vi "array -- bilinear regression 3D -- V3.vi"(7 "action":T3, 9 "fit map IN":map{T2, dbl}(c390), 11 "xyzw IN":T1={"x"=[-2.0, -1.0, 0.0, 1.0, 2.0], "y"=[-2.0, -1.0, 0.0, 1.0, 2.0], "w"=[-2.0, -1.0, 0.0, 1.0, 2.0], "z"=[12.0, 3.0, 0.0, 3.0, 12.0]}) -> (1 "fit map out":map{T2, dbl}(c390), 3 "xyzw OUT":T1={"x"=[-2.0, -1.0, 0.0, 1.0, 2.0], "y"=[-2.0, -1.0, 0.0, 1.0, 2.0], "w"=[-2.0, -1.0, 0.0, 1.0, 2.0], "z"=[12.0, 3.0, 0.0, 3.0, 12.0]})   [LabVIEW 2021]
uses:
  array -- fit control .ctl
  array -- bilinear regression 2D.ctl
  4-vec-array.ctl
  <vilib>/Analysis/baseanly.llb/Matrix Type of Inverse Matrix.ctl
  <vilib>/Analysis/7linalg.llb/Solve Linear Equations (single right hand).vi
  <vilib>/Analysis/baseanly.llb/Real A x B.vi
  <vilib>/Analysis/baseanly.llb/Solve Linear Equations By Cholesky.vi
  <vilib>/Analysis/baseanly.llb/Real Matrix to Compact Array.vi
  <vilib>/Analysis/baseanly.llb/Real Compact Tri-Matrix Linear Eqs.vi
  <vilib>/Analysis/Matrix/Numeric/Conversions/Array To Matrix - RA2.vi
  <vilib>/Analysis/7linalg.llb/Solve Linear Eqs (General).vi
  <vilib>/Analysis/7linalg.llb/Solve Linear Eqs (Gen, single right hand).vi
  <vilib>/Analysis/Matrix/Numeric/Conversions/Matrix To Array - RM.vi
  <vilib>/Analysis/NI_AALBase.lvlib
  <vilib>/Analysis/Matrix/NI_Matrix.lvlib
  <vilib>/Analysis/NI_AALPro.lvlib
panel:
  out "fit  IN":dbl[](array[numeric])=[1.9, 2.6, 3.3, 1.0, 2.7, 3.9]
  out "fit OUT":dbl[](array[numeric])=[1.0, 1.0, 1.0, 0.0, 0.0, 0.0]
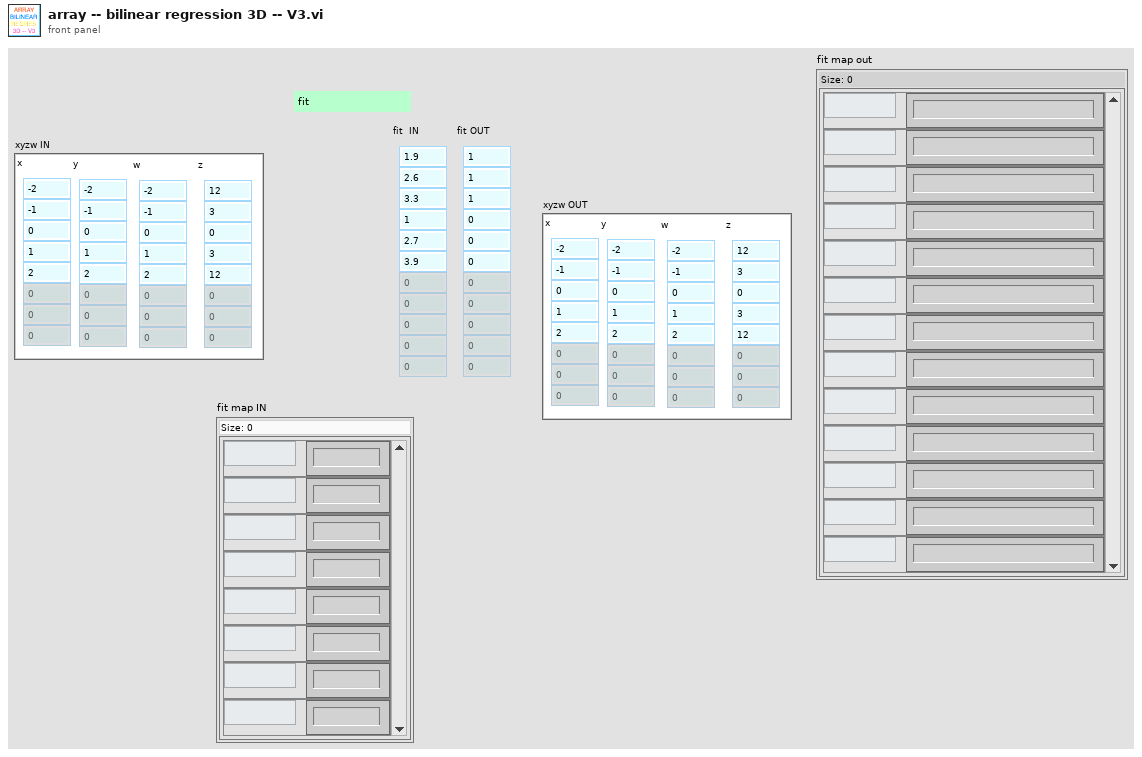
[diagram p1: front panel]
types:
  T1 = typedef "4-vec-array.ctl" = cluster{"x":dbl[], "y":dbl[], "w":dbl[], "z":dbl[]}
  T2 = typedef "array -- bilinear regression 2D.ctl" = enum16{"1", "x", "y", "xx", "xy", "yy", "xxy", "xyy", "yyy", "xxx", "xxyy", "xyyy", "xxxy", "yyyy", "xxxx", "xxz", "xyz", "yyz", "xz", "yz", "z", "wwz", "ywz", "xwz", "xxxw", "xxyw", "xyyw", "yyyw", "xxww", "xyww", "yyww", "xwww", "ywww", "wwww", "ww", "xw", "yw", "w", "wz", "xxw", "yyw", "xyw", "xww", "yww", "www"}
  T3 = typedef "array -- fit control .ctl" = enum16{"fit", "calc", "check", "init"}
  T4 = typedef "NI_AALBase.lvlib/Matrix Type of Inverse Matrix.ctl" = enum32{"General", "Positive Definite", "Lower Triangular", "Upper Triangular"}
  T5 = typedef "NI_Matrix.lvlib/RealMatrix.ctl" = dbl[][]
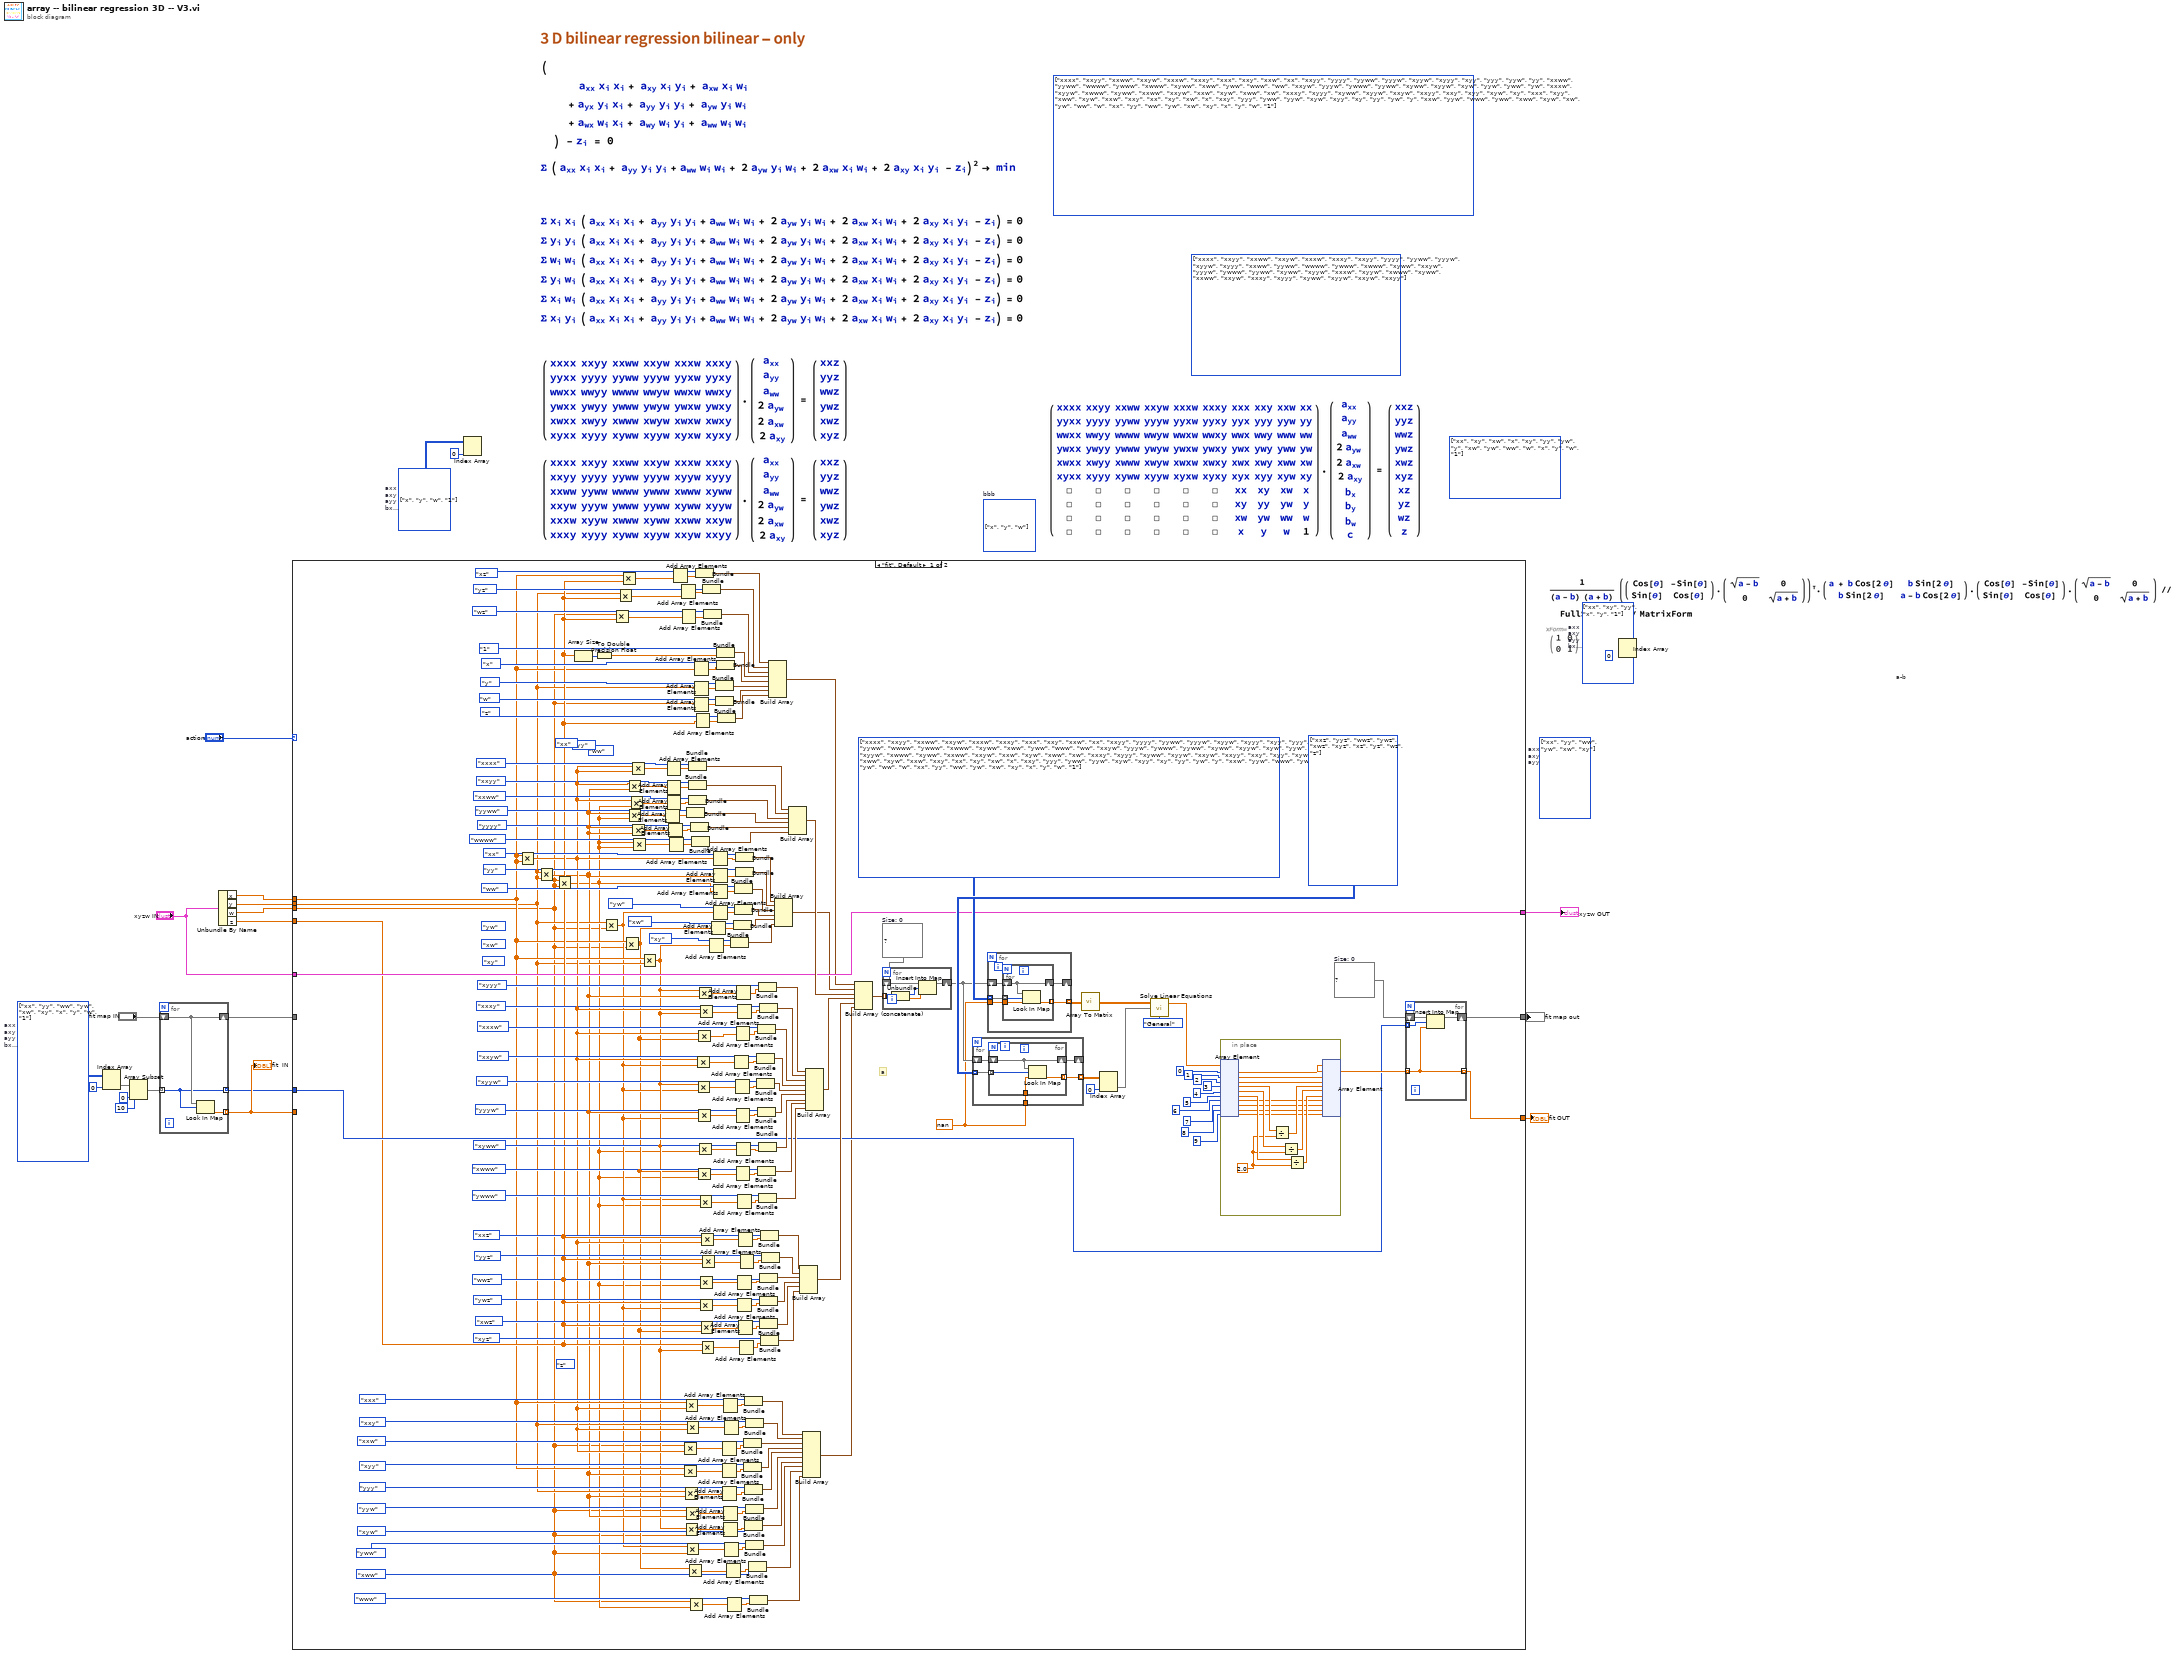
[diagram p0: block diagram]
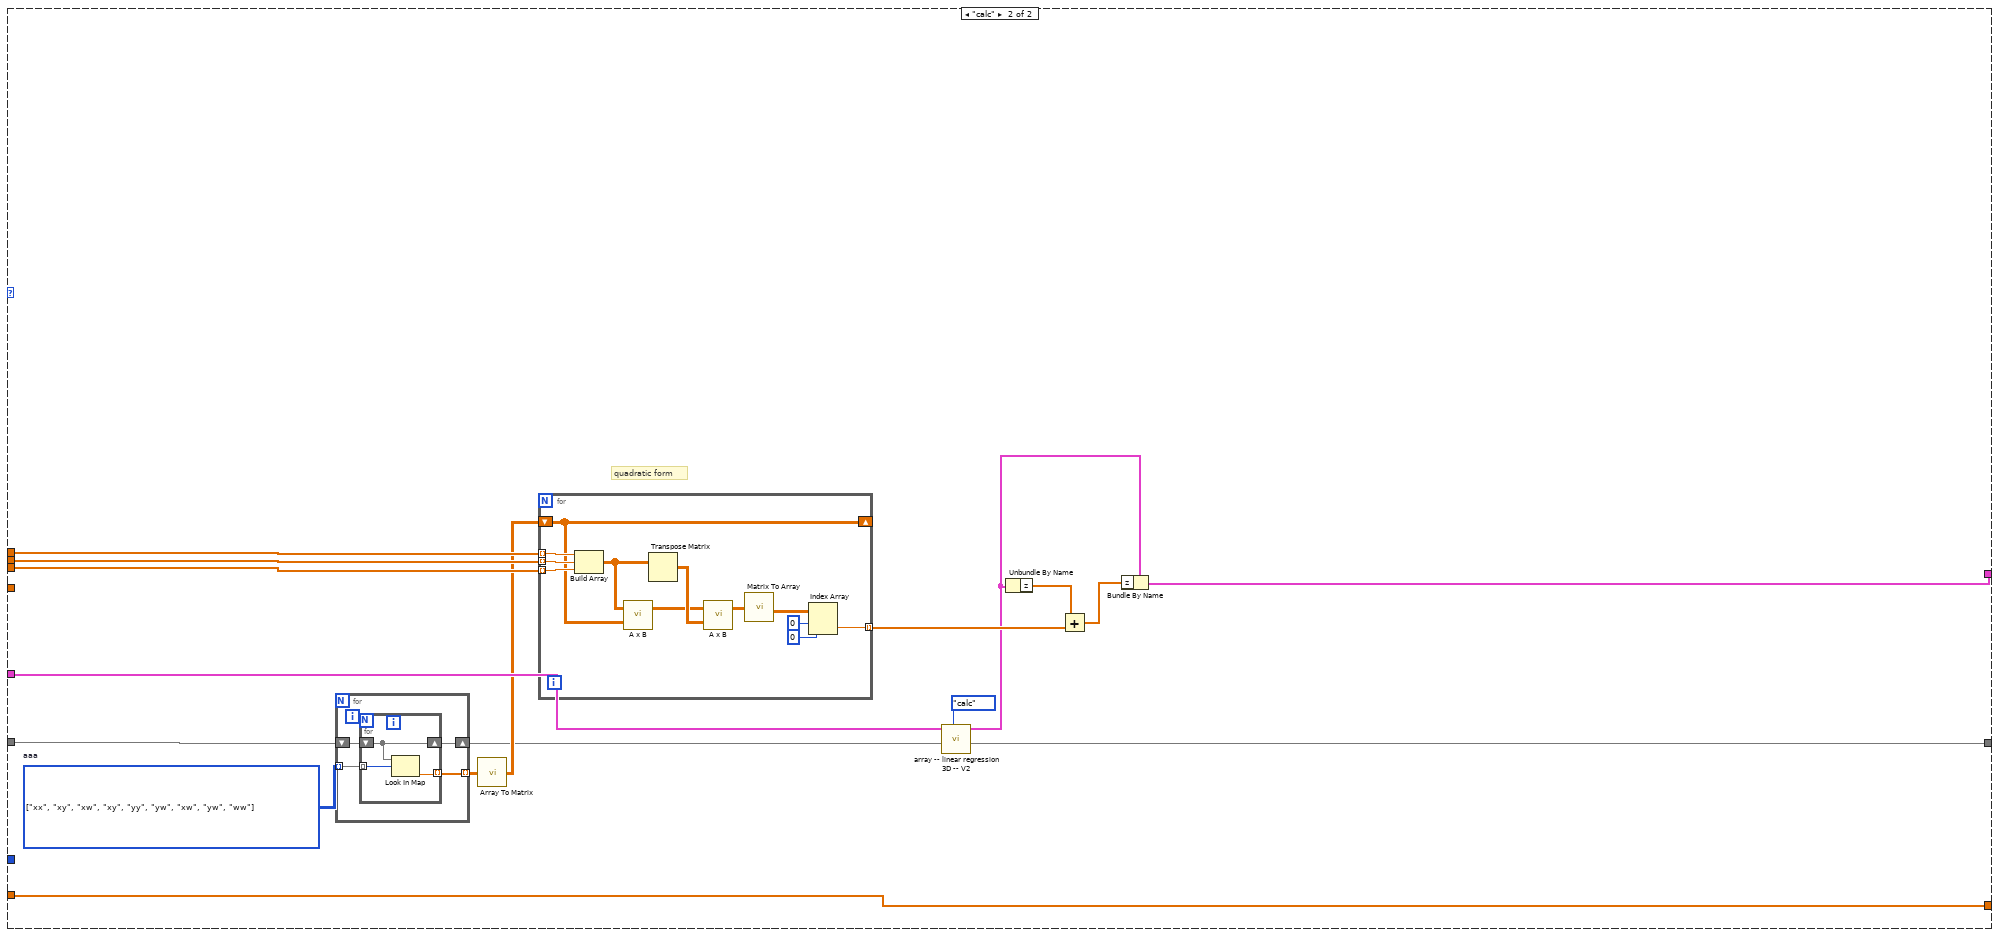
[diagram p2: hidden frame]
diagram:
  (unwired) T2[][] [[enum."xxxx", enum."xxyy", enum."xxww", enum."xxyw", enum."xxxw", enum."xxxy", enum."xxx", enum."xxy", enum."xxw", enum."xx"], [enum."xxyy", enum."yyyy", enum."yyww", enum."yyyw", enum."xyyw", enum."xyyy", enum."xyy", enum."yyy", enum."yyw", enum."yy"], [enum."xxww", enum."yyww", enum."wwww", enum."ywww", enum."xwww", enum."xyww", enum."xww", enum."yww", enum."www", enum."ww"], [enum."xxyw", enum."yyyw", enum."ywww", enum."yyww", enum."xyww", enum."xyyw", enum."xyw", enum."yyw", enum."yww", enum."yw"], [enum."xxxw", enum."xyyw", enum."xwww", enum."xyww", enum."xxww", enum."xxyw", enum."xxw", enum."xyw", enum."xww", enum."xw"], [enum."xxxy", enum."xyyy", enum."xyww", enum."xyyw", enum."xxyw", enum."xxyy", enum."xxy", enum."xyy", enum."xyw", enum."xy"], [enum."xxx", enum."xyy", enum."xww", enum."xyw", enum."xxw", enum."xxy", enum."xx", enum."xy", enum."xw", enum."x"], [enum."xxy", enum."yyy", enum."yww", enum."yyw", enum."xyw", enum."xyy", enum."xy", enum."yy", enum."yw", enum."y"], [enum."xxw", enum."yyw", enum."www", enum."yww", enum."xww", enum."xyw", enum."xw", enum."yw", enum."ww", enum."w"], [enum."xx", enum."yy", enum."ww", enum."yw", enum."xw", enum."xy", enum."x", enum."y", enum."w", enum."1"]] items=["1", "x", "y", "xx", "xy", "yy", "xxy", "xyy", "yyy", "xxx", "xxyy", "xyyy", "xxxy", "yyyy", "xxxx", "xxz", "xyz", "yyz", "xz", "yz", "z", "wwz", "ywz", "xwz", "xxxw", "xxyw", "xyyw", "yyyw", "xxww", "xyww", "yyww", "xwww", "ywww", "wwww", "ww", "xw", "yw", "w", "wz", "xxw", "yyw", "xyw", "xww", "yww", "www"]
  (unwired) T2[][] [[enum."xxxx", enum."xxyy", enum."xxww", enum."xxyw", enum."xxxw", enum."xxxy"], [enum."xxyy", enum."yyyy", enum."yyww", enum."yyyw", enum."xyyw", enum."xyyy"], [enum."xxww", enum."yyww", enum."wwww", enum."ywww", enum."xwww", enum."xyww"], [enum."xxyw", enum."yyyw", enum."ywww", enum."yyww", enum."xyww", enum."xyyw"], [enum."xxxw", enum."xyyw", enum."xwww", enum."xyww", enum."xxww", enum."xxyw"], [enum."xxxy", enum."xyyy", enum."xyww", enum."xyyw", enum."xxyw", enum."xxyy"]] items=["1", "x", "y", "xx", "xy", "yy", "xxy", "xyy", "yyy", "xxx", "xxyy", "xyyy", "xxxy", "yyyy", "xxxx", "xxz", "xyz", "yyz", "xz", "yz", "z", "wwz", "ywz", "xwz", "xxxw", "xxyw", "xyyw", "yyyw", "xxww", "xyww", "yyww", "xwww", "ywww", "wwww", "ww", "xw", "yw", "w", "wz", "xxw", "yyw", "xyw", "xww", "yww", "www"]
  (unwired) T2[][] [[enum."xx", enum."xy", enum."xw", enum."x"], [enum."xy", enum."yy", enum."yw", enum."y"], [enum."xw", enum."yw", enum."ww", enum."w"], [enum."x", enum."y", enum."w", enum."1"]] items=["1", "x", "y", "xx", "xy", "yy", "xxy", "xyy", "yyy", "xxx", "xxyy", "xyyy", "xxxy", "yyyy", "xxxx", "xxz", "xyz", "yyz", "xz", "yz", "z", "wwz", "ywz", "xwz", "xxxw", "xxyw", "xyyw", "yyyw", "xxww", "xyww", "yyww", "xwww", "ywww", "wwww", "ww", "xw", "yw", "w", "wz", "xxw", "yyw", "xyw", "xww", "yww", "www"]
  (unwired) T2[][] [[enum."xx"], [enum."yy"], [enum."ww"], [enum."yw"], [enum."xw"], [enum."xy"]] items=["1", "x", "y", "xx", "xy", "yy", "xxy", "xyy", "yyy", "xxx", "xxyy", "xyyy", "xxxy", "yyyy", "xxxx", "xxz", "xyz", "yyz", "xz", "yz", "z", "wwz", "ywz", "xwz", "xxxw", "xxyw", "xyyw", "yyyw", "xxww", "xyww", "yyww", "xwww", "ywww", "wwww", "ww", "xw", "yw", "w", "wz", "xxw", "yyw", "xyw", "xww", "yww", "www"]  # axx axy ayy
  (unwired) T2[][] [[enum."x"], [enum."y"], [enum."w"]] items=["1", "x", "y", "xx", "xy", "yy", "xxy", "xyy", "yyy", "xxx", "xxyy", "xyyy", "xxxy", "yyyy", "xxxx", "xxz", "xyz", "yyz", "xz", "yz", "z", "wwz", "ywz", "xwz", "xxxw", "xxyw", "xyyw", "yyyw", "xxww", "xyww", "yyww", "xwww", "ywww", "wwww", "ww", "xw", "yw", "w", "wz", "xxw", "yyw", "xyw", "xww", "yww", "www"]  # bbb
  w17 = T2[][] [[enum."x"], [enum."y"], [enum."w"], [enum."1"]] items=["1", "x", "y", "xx", "xy", "yy", "xxy", "xyy", "yyy", "xxx", "xxyy", "xyyy", "xxxy", "yyyy", "xxxx", "xxz", "xyz", "yyz", "xz", "yz", "z", "wwz", "ywz", "xwz", "xxxw", "xxyw", "xyyw", "yyyw", "xxww", "xyww", "yyww", "xwww", "ywww", "wwww", "ww", "xw", "yw", "w", "wz", "xxw", "yyw", "xyw", "xww", "yww", "www"]  # axx axy ayy bx by c
  w19 = T2[][] [[enum."xx"], [enum."yy"], [enum."ww"], [enum."yw"], [enum."xw"], [enum."xy"], [enum."x"], [enum."y"], [enum."w"], [enum."1"]] items=["1", "x", "y", "xx", "xy", "yy", "xxy", "xyy", "yyy", "xxx", "xxyy", "xyyy", "xxxy", "yyyy", "xxxx", "xxz", "xyz", "yyz", "xz", "yz", "z", "wwz", "ywz", "xwz", "xxxw", "xxyw", "xyyw", "yyyw", "xxww", "xyww", "yyww", "xwww", "ywww", "wwww", "ww", "xw", "yw", "w", "wz", "xxw", "yyw", "xyw", "xww", "yww", "www"]  # axx axy ayy bx by c
  w21 = T2[][] [[enum."xx"], [enum."xy"], [enum."yy"], [enum."x"], [enum."y"], [enum."1"]] items=["1", "x", "y", "xx", "xy", "yy", "xxy", "xyy", "yyy", "xxx", "xxyy", "xyyy", "xxxy", "yyyy", "xxxx", "xxz", "xyz", "yyz", "xz", "yz", "z", "wwz", "ywz", "xwz", "xxxw", "xxyw", "xyyw", "yyyw", "xxww", "xyww", "yyww", "xwww", "ywww", "wwww", "ww", "xw", "yw", "w", "wz", "xxw", "yyw", "xyw", "xww", "yww", "www"]  # axx axy ayy bx by c
  # "a-b"
  n1 = Index Array(array=w19, index (col)=0 ("disabled index (col)")) -> (element=w15:T2[])  [unwired: 1 in]
  n2 = Array Subset(array=w15, index=0, length=10) -> (w9:T2[])
  n3 = for {
    shift-right: [w25] -> w8
    shift-left: "fit map IN" -> [w25]
    tunnel: w9 -> [w24] mode=indexing
    tunnel: [w26] -> w10 mode=indexing
    tunnel: [w24] -> w7 mode=indexing
    n4 = Look In Map(map=w25, key=w24) -> (value=w26:dbl)  [unwired: 1 in, 1 out]
  }
  "fit  IN" <- w10
  n5 = Unbundle By Name("xyzw IN") -> ("x"=w4:dbl[], "y"=w3:dbl[], "w"=w2:dbl[], "z"=w1:dbl[])
  n6 = case shown="\"fit\", Default" "action" {
    tunnel: w1 -> [w85 _]
    tunnel: w4 -> [w42 w295]
    tunnel: [w141 w289] -> w22
    tunnel: w3 -> [w40 w294]
    tunnel: w2 -> [w34 w293]
    tunnel: w8 -> [_ w290]
    tunnel: "xyzw IN" -> [w144 w298]
    tunnel: [w144 w283] -> w6
    tunnel: [w145 w287] -> w12
    tunnel: w10 -> [_ w289]
    tunnel: w7 -> [w143 _]
    frame "fit", Default {
      (unwired) array_--_bilinear_regression_2D."z"
      w132 = nan ("default value")
      (unwired) array_--_bilinear_regression_2D."ww"
      (unwired) array_--_bilinear_regression_2D."yy"
      (unwired) array_--_bilinear_regression_2D."xx"
      w28 = map{T2, dbl} {}  # Size: 0
      w227 = T2[][] [[enum."xxz"], [enum."yyz"], [enum."wwz"], [enum."ywz"], [enum."xwz"], [enum."xyz"], [enum."xz"], [enum."yz"], [enum."wz"], [enum."z"]] items=["1", "x", "y", "xx", "xy", "yy", "xxy", "xyy", "yyy", "xxx", "xxyy", "xyyy", "xxxy", "yyyy", "xxxx", "xxz", "xyz", "yyz", "xz", "yz", "z", "wwz", "ywz", "xwz", "xxxw", "xxyw", "xyyw", "yyyw", "xxww", "xyww", "yyww", "xwww", "ywww", "wwww", "ww", "xw", "yw", "w", "wz", "xxw", "yyw", "xyw", "xww", "yww", "www"]
      w226 = T2[][] [[enum."xxxx", enum."xxyy", enum."xxww", enum."xxyw", enum."xxxw", enum."xxxy", enum."xxx", enum."xxy", enum."xxw", enum."xx"], [enum."xxyy", enum."yyyy", enum."yyww", enum."yyyw", enum."xyyw", enum."xyyy", enum."xyy", enum."yyy", enum."yyw", enum."yy"], [enum."xxww", enum."yyww", enum."wwww", enum."ywww", enum."xwww", enum."xyww", enum."xww", enum."yww", enum."www", enum."ww"], [enum."xxyw", enum."yyyw", enum."ywww", enum."yyww", enum."xyww", enum."xyyw", enum."xyw", enum."yyw", enum."yww", enum."yw"], [enum."xxxw", enum."xyyw", enum."xwww", enum."xyww", enum."xxww", enum."xxyw", enum."xxw", enum."xyw", enum."xww", enum."xw"], [enum."xxxy", enum."xyyy", enum."xyww", enum."xyyw", enum."xxyw", enum."xxyy", enum."xxy", enum."xyy", enum."xyw", enum."xy"], [enum."xxx", enum."xyy", enum."xww", enum."xyw", enum."xxw", enum."xxy", enum."xx", enum."xy", enum."xw", enum."x"], [enum."xxy", enum."yyy", enum."yww", enum."yyw", enum."xyw", enum."xyy", enum."xy", enum."yy", enum."yw", enum."y"], [enum."xxw", enum."yyw", enum."www", enum."yww", enum."xww", enum."xyw", enum."xw", enum."yw", enum."ww", enum."w"], [enum."xx", enum."yy", enum."ww", enum."yw", enum."xw", enum."xy", enum."x", enum."y", enum."w", enum."1"]] items=["1", "x", "y", "xx", "xy", "yy", "xxy", "xyy", "yyy", "xxx", "xxyy", "xyyy", "xxxy", "yyyy", "xxxx", "xxz", "xyz", "yyz", "xz", "yz", "z", "wwz", "ywz", "xwz", "xxxw", "xxyw", "xyyw", "yyyw", "xxww", "xyww", "yyww", "xwww", "ywww", "wwww", "ww", "xw", "yw", "w", "wz", "xxw", "yyw", "xyw", "xww", "yww", "www"]
      w229 = map{T2, dbl} {}  # Size: 0
      (unwired) array_--_bilinear_regression_2D."xy"
      (unwired) array_--_bilinear_regression_2D."xw"
      (unwired) array_--_bilinear_regression_2D."yw"
      # "a"
      n7 = Multiply(x=w42, y=w42) -> (x*y=w41:dbl[])
      n8 = Multiply(x=w40, y=w40) -> (x*y=w39:dbl[])
      n9 = Multiply(x=w34, y=w34) -> (x*y=w35:dbl[])
      n10 = Array Size(array=w85) -> (size(s)=w108:i32)
      n11 = To Double Precision Float(number=w108) -> (double precision float=w107:dbl)
      n12 = Multiply(x=w40, y=w34) -> (x*y=w37:dbl[])
      n13 = Multiply(x=w34, y=w85) -> (x*y=w84:dbl[])
      n14 = Multiply(x=w40, y=w85) -> (x*y=w83:dbl[])
      n15 = Multiply(x=w42, y=w85) -> (x*y=w82:dbl[])
      n16 = Multiply(x=w42, y=w34) -> (x*y=w36:dbl[])
      n17 = Multiply(x=w41, y=w39) -> (x*y=w222:dbl[])
      n18 = Multiply(x=w39, y=w35) -> (x*y=w219:dbl[])
      n19 = Multiply(x=w41, y=w35) -> (x*y=w221:dbl[])
      n20 = Multiply(x=w41, y=w41) -> (x*y=w240:dbl[])
      n21 = Multiply(x=w39, y=w39) -> (x*y=w217:dbl[])
      n22 = Multiply(x=w35, y=w35) -> (x*y=w215:dbl[])
      n23 = Multiply(x=w42, y=w40) -> (x*y=w38:dbl[])
      n24 = Add Array Elements(numeric array=w219) -> (sum=w220:dbl)
      n25 = Add Array Elements(numeric array=w240) -> (sum=w239:dbl)
      n26 = Add Array Elements(numeric array=w222) -> (sum=w237:dbl)
      n27 = Add Array Elements(numeric array=w221) -> (sum=w234:dbl)
      n28 = Add Array Elements(numeric array=w217) -> (sum=w218:dbl)
      n29 = Add Array Elements(numeric array=w215) -> (sum=w216:dbl)
      n30 = Add Array Elements(numeric array=w82) -> (sum=w91:dbl)
      n31 = Add Array Elements(numeric array=w83) -> (sum=w90:dbl)
      n32 = Add Array Elements(numeric array=w84) -> (sum=w89:dbl)
      n33 = Multiply(x=w34, y=w41) -> (x*y=w71:dbl[])
      n34 = Multiply(x=w42, y=w39) -> (x*y=w73:dbl[])
      n35 = Multiply(x=w40, y=w39) -> (x*y=w75:dbl[])
      n36 = Multiply(x=w42, y=w41) -> (x*y=w67:dbl[])
      n37 = Multiply(x=w38, y=w34) -> (x*y=w51:dbl[])
      n38 = Multiply(x=w34, y=w39) -> (x*y=w77:dbl[])
      n39 = Multiply(x=w40, y=w41) -> (x*y=w69:dbl[])
      n40 = Multiply(x=w37, y=w34) -> (x*y=w53:dbl[])
      n41 = Multiply(x=w36, y=w34) -> (x*y=w47:dbl[])
      n42 = Bundle(array_--_bilinear_regression_2D."yyww", "Numeric"=w220) -> (w214:cluster{T2, "Numeric":dbl})  [unwired: 1 in]
      n43 = Multiply(x=w34, y=w35) -> (x*y=w49:dbl[])
      n44 = Bundle(array_--_bilinear_regression_2D."xxxx", "Numeric"=w239) -> (w223:cluster{T2, "Numeric":dbl})  [unwired: 1 in]
      n45 = Bundle(array_--_bilinear_regression_2D."xxyy", "Numeric"=w237) -> (w224:cluster{T2, "Numeric":dbl})  [unwired: 1 in]
      n46 = Bundle(array_--_bilinear_regression_2D."xxww", "Numeric"=w234) -> (w225:cluster{T2, "Numeric":dbl})  [unwired: 1 in]
      n47 = Bundle(array_--_bilinear_regression_2D."yyyy", "Numeric"=w218) -> (w210:cluster{T2, "Numeric":dbl})  [unwired: 1 in]
      n48 = Bundle(array_--_bilinear_regression_2D."wwww", "Numeric"=w216) -> (w209:cluster{T2, "Numeric":dbl})  [unwired: 1 in]
      n49 = Add Array Elements(numeric array=w40) -> (sum=w114:dbl)
      n50 = Add Array Elements(numeric array=w34) -> (sum=w113:dbl)
      n51 = Add Array Elements(numeric array=w42) -> (sum=w115:dbl)
      n52 = Add Array Elements(numeric array=w85) -> (sum=w106:dbl)
      n53 = Multiply(x=w41, y=w37) -> (x*y=w203:dbl[])
      n54 = Multiply(x=w38, y=w37) -> (x*y=w201:dbl[])
      n55 = Bundle(array_--_bilinear_regression_2D."xz", "Numeric"=w91) -> (w81:cluster{T2, "Numeric":dbl})  [unwired: 1 in]
      n56 = Multiply(x=w41, y=w36) -> (x*y=w205:dbl[])
      n57 = Multiply(x=w39, y=w37) -> (x*y=w199:dbl[])
      n58 = Multiply(x=w36, y=w35) -> (x*y=w195:dbl[])
      n59 = Multiply(x=w38, y=w39) -> (x*y=w241:dbl[])
      n60 = Multiply(x=w38, y=w35) -> (x*y=w197:dbl[])
      n61 = Multiply(x=w37, y=w35) -> (x*y=w193:dbl[])
      n62 = Multiply(x=w41, y=w38) -> (x*y=w207:dbl[])
      n63 = Multiply(x=w85, y=w35) -> (x*y=w165:dbl[])
      n64 = Multiply(x=w85, y=w37) -> (x*y=w167:dbl[])
      n65 = Multiply(x=w85, y=w36) -> (x*y=w169:dbl[])
      n66 = Multiply(x=w85, y=w41) -> (x*y=w161:dbl[])
      n67 = Multiply(x=w85, y=w38) -> (x*y=w171:dbl[])
      n68 = Multiply(x=w85, y=w39) -> (x*y=w163:dbl[])
      n69 = Bundle(array_--_bilinear_regression_2D."yz", "Numeric"=w90) -> (w80:cluster{T2, "Numeric":dbl})  [unwired: 1 in]
      n70 = Bundle(array_--_bilinear_regression_2D."wz", "Numeric"=w89) -> (w79:cluster{T2, "Numeric":dbl})  [unwired: 1 in]
      n71 = Add Array Elements(numeric array=w38) -> (sum=w121:dbl)
      n72 = Add Array Elements(numeric array=w36) -> (sum=w122:dbl)
      n73 = Add Array Elements(numeric array=w35) -> (sum=w124:dbl)
      n74 = Add Array Elements(numeric array=w37) -> (sum=w123:dbl)
      n75 = Add Array Elements(numeric array=w41) -> (sum=w127:dbl)
      n76 = Add Array Elements(numeric array=w39) -> (sum=w125:dbl)
      n77 = Bundle(array_--_bilinear_regression_2D."y", "Numeric"=w114) -> (w102:cluster{T2, "Numeric":dbl})  [unwired: 1 in]
      n78 = Bundle(array_--_bilinear_regression_2D."w", "Numeric"=w113) -> (w101:cluster{T2, "Numeric":dbl})  [unwired: 1 in]
      n79 = Bundle(array_--_bilinear_regression_2D."1", w107) -> (w104:cluster{T2, dbl})  [unwired: 1 in]
      n80 = Bundle(array_--_bilinear_regression_2D."x", "Numeric"=w115) -> (w103:cluster{T2, "Numeric":dbl})  [unwired: 1 in]
      n81 = Bundle(array_--_bilinear_regression_2D."z", "Numeric"=w106) -> (w100:cluster{T2, "Numeric":dbl})  [unwired: 1 in]
      n82 = Add Array Elements(numeric array=w71) -> (sum=w72:dbl)
      n83 = Add Array Elements(numeric array=w73) -> (sum=w74:dbl)
      n84 = Add Array Elements(numeric array=w75) -> (sum=w76:dbl)
      n85 = Add Array Elements(numeric array=w67) -> (sum=w68:dbl)
      n86 = Add Array Elements(numeric array=w51) -> (sum=w52:dbl)
      n87 = Add Array Elements(numeric array=w77) -> (sum=w78:dbl)
      n88 = Add Array Elements(numeric array=w69) -> (sum=w70:dbl)
      n89 = Add Array Elements(numeric array=w53) -> (sum=w54:dbl)
      n90 = Add Array Elements(numeric array=w47) -> (sum=w48:dbl)
      n91 = Add Array Elements(numeric array=w49) -> (sum=w50:dbl)
      n92 = Bundle(array_--_bilinear_regression_2D."xy", "Numeric"=w121) -> (w94:cluster{T2, "Numeric":dbl})  [unwired: 1 in]
      n93 = Add Array Elements(numeric array=w203) -> (sum=w204:dbl)
      n94 = Bundle(array_--_bilinear_regression_2D."xw", "Numeric"=w122) -> (w95:cluster{T2, "Numeric":dbl})  [unwired: 1 in]
      n95 = Add Array Elements(numeric array=w201) -> (sum=w202:dbl)
      n96 = Add Array Elements(numeric array=w205) -> (sum=w206:dbl)
      n97 = Add Array Elements(numeric array=w199) -> (sum=w200:dbl)
      n98 = Add Array Elements(numeric array=w195) -> (sum=w196:dbl)
      n99 = Add Array Elements(numeric array=w241) -> (sum=w232:dbl)
      n100 = Add Array Elements(numeric array=w197) -> (sum=w198:dbl)
      n101 = Bundle(array_--_bilinear_regression_2D."ww", "Numeric"=w124) -> (w97:cluster{T2, "Numeric":dbl})  [unwired: 1 in]
      n102 = Bundle(array_--_bilinear_regression_2D."yw", "Numeric"=w123) -> (w96:cluster{T2, "Numeric":dbl})  [unwired: 1 in]
      n103 = Add Array Elements(numeric array=w193) -> (sum=w194:dbl)
      n104 = Bundle(array_--_bilinear_regression_2D."xx", "Numeric"=w127) -> (w99:cluster{T2, "Numeric":dbl})  [unwired: 1 in]
      n105 = Bundle(array_--_bilinear_regression_2D."yy", "Numeric"=w125) -> (w98:cluster{T2, "Numeric":dbl})  [unwired: 1 in]
      n106 = Add Array Elements(numeric array=w207) -> (sum=w208:dbl)
      n107 = Add Array Elements(numeric array=w165) -> (sum=w166:dbl)
      n108 = Add Array Elements(numeric array=w167) -> (sum=w168:dbl)
      n109 = Add Array Elements(numeric array=w169) -> (sum=w170:dbl)
      n110 = Add Array Elements(numeric array=w161) -> (sum=w162:dbl)
      n111 = Add Array Elements(numeric array=w171) -> (sum=w172:dbl)
      n112 = Add Array Elements(numeric array=w163) -> (sum=w164:dbl)
      n113 = Bundle(array_--_bilinear_regression_2D."xxw", "Numeric"=w72) -> (w64:cluster{T2, "Numeric":dbl})  [unwired: 1 in]
      n114 = Bundle(array_--_bilinear_regression_2D."xyy", "Numeric"=w74) -> (w63:cluster{T2, "Numeric":dbl})  [unwired: 1 in]
      n115 = Bundle(array_--_bilinear_regression_2D."yyy", "Numeric"=w76) -> (w62:cluster{T2, "Numeric":dbl})  [unwired: 1 in]
      n116 = Bundle(array_--_bilinear_regression_2D."xxx", "Numeric"=w68) -> (w66:cluster{T2, "Numeric":dbl})  [unwired: 1 in]
      n117 = Bundle(array_--_bilinear_regression_2D."xyw", "Numeric"=w52) -> (w33:cluster{T2, "Numeric":dbl})  [unwired: 1 in]
      n118 = Bundle(array_--_bilinear_regression_2D."yyw", "Numeric"=w78) -> (w61:cluster{T2, "Numeric":dbl})  [unwired: 1 in]
      n119 = Bundle(array_--_bilinear_regression_2D."xxy", "Numeric"=w70) -> (w65:cluster{T2, "Numeric":dbl})  [unwired: 1 in]
      n120 = Bundle(array_--_bilinear_regression_2D."yww", "Numeric"=w54) -> (w32:cluster{T2, "Numeric":dbl})  [unwired: 1 in]
      n121 = Bundle(array_--_bilinear_regression_2D."xww", "Numeric"=w48) -> (w31:cluster{T2, "Numeric":dbl})  [unwired: 1 in]
      n122 = Bundle(array_--_bilinear_regression_2D."www", "Numeric"=w50) -> (w30:cluster{T2, "Numeric":dbl})  [unwired: 1 in]
      n123 = Bundle(array_--_bilinear_regression_2D."xxyw", "Numeric"=w204) -> (w178:cluster{T2, "Numeric":dbl})  [unwired: 1 in]
      n124 = Bundle(array_--_bilinear_regression_2D."xyyw", "Numeric"=w202) -> (w177:cluster{T2, "Numeric":dbl})  [unwired: 1 in]
      n125 = Bundle(array_--_bilinear_regression_2D."xxxw", "Numeric"=w206) -> (w179:cluster{T2, "Numeric":dbl})  [unwired: 1 in]
      n126 = Bundle(array_--_bilinear_regression_2D."yyyw", "Numeric"=w200) -> (w176:cluster{T2, "Numeric":dbl})  [unwired: 1 in]
      n127 = Bundle(array_--_bilinear_regression_2D."xwww", "Numeric"=w196) -> (w174:cluster{T2, "Numeric":dbl})  [unwired: 1 in]
      n128 = Bundle(array_--_bilinear_regression_2D."xyyy", "Numeric"=w232) -> (w181:cluster{T2, "Numeric":dbl})  [unwired: 1 in]
      n129 = Bundle(array_--_bilinear_regression_2D."xyww", "Numeric"=w198) -> (w175:cluster{T2, "Numeric":dbl})  [unwired: 1 in]
      n130 = Bundle(array_--_bilinear_regression_2D."ywww", "Numeric"=w194) -> (w173:cluster{T2, "Numeric":dbl})  [unwired: 1 in]
      n131 = Bundle(array_--_bilinear_regression_2D."xxxy", "Numeric"=w208) -> (w180:cluster{T2, "Numeric":dbl})  [unwired: 1 in]
      n132 = Bundle(array_--_bilinear_regression_2D."wwz", "Numeric"=w166) -> (w158:cluster{T2, "Numeric":dbl})  [unwired: 1 in]
      n133 = Bundle(array_--_bilinear_regression_2D."ywz", "Numeric"=w168) -> (w157:cluster{T2, "Numeric":dbl})  [unwired: 1 in]
      n134 = Bundle(array_--_bilinear_regression_2D."xwz", "Numeric"=w170) -> (w156:cluster{T2, "Numeric":dbl})  [unwired: 1 in]
      n135 = Bundle(array_--_bilinear_regression_2D."xxz", "Numeric"=w162) -> (w160:cluster{T2, "Numeric":dbl})  [unwired: 1 in]
      n136 = Bundle(array_--_bilinear_regression_2D."xyz", "Numeric"=w172) -> (w155:cluster{T2, "Numeric":dbl})  [unwired: 1 in]
      n137 = Bundle(array_--_bilinear_regression_2D."yyz", "Numeric"=w164) -> (w159:cluster{T2, "Numeric":dbl})  [unwired: 1 in]
      n138 = Build Array(w81, w80, w79, w104, w103, w102, w101, w100) -> (w93:cluster{T2, "Numeric":dbl}[])
      n139 = Build Array(w99, w98, w97, w96, w95, w94) -> (w92:cluster{T2, "Numeric":dbl}[])
      n140 = Build Array(w223, w224, w225, w214, w210, w209) -> (w183:cluster{T2, "Numeric":dbl}[])
      n141 = Build Array(w160, w159, w158, w157, w156, w155) -> (w148:cluster{T2, "Numeric":dbl}[])
      n142 = Build Array(w66, w65, w64, w63, w62, w61, w33, w32, w31, w30) -> (w29:cluster{T2, "Numeric":dbl}[])
      n143 = Build Array(w181, w180, w179, w178, w177, w176, w175, w174, w173) -> (w182:cluster{T2, "Numeric":dbl}[])
      n144 = Build Array (concatenate)(w93, w92, w183, w182, w148, w29) -> (w184:cluster{T2, "Numeric":dbl}[])
      n145 = for {
        tunnel: w184 -> [w271] mode=indexing
        shift-right: [w272] -> w142
        shift-left: w229 -> [w273]
        n146 = Unbundle(w271) -> (w270:T2, "Numeric"=w269:dbl)
        n147 = Insert Into Map(map in=w273, key=w270, value=w269) -> (map out=w272:map{T2, dbl})  [unwired: 2 out]
      }
      n148 = for {
        shift-right: [w263] -> _
        shift-left: w142 -> [w264]
        tunnel: w227 -> [w262] mode=indexing
        tunnel: [w261] -> w137 mode=indexing
        tunnel: w132 -> [w260]
        n149 = for {
          shift-right: [w268] -> w263
          shift-left: w264 -> [w268]
          tunnel: w262 -> [w267] mode=indexing
          tunnel: [w266] -> w261 mode=indexing
          tunnel: w260 -> [w265]
          n150 = Look In Map(map=w268, key=w267, default value=w265) -> (value=w266:dbl)  [unwired: 1 out]
        }
      }
      n151 = for {
        tunnel: w226 -> [w278] mode=indexing
        shift-right: [w276] -> _
        shift-left: w142 -> [w277]
        tunnel: [w275] -> w231 mode=indexing
        tunnel: w132 -> [w274]
        n152 = for {
          tunnel: w278 -> [w281] mode=indexing
          shift-right: [w282] -> w276
          shift-left: w277 -> [w282]
          tunnel: [w280] -> w275 mode=indexing
          tunnel: w274 -> [w279]
          n153 = Look In Map(map=w282, key=w281, default value=w279) -> (value=w280:dbl)  [unwired: 1 out]
        }
      }
      n154 = call-poly <vilib>:"Array To Matrix.vi"("Real 2D Array"=w231) -> ("Real Matrix"=w27:T5)
      n155 = Index Array(array=w137, index (col)=0 ("disabled index (col)")) -> (element=w139:dbl[])  [unwired: 1 in]
      n156 = call-poly <vilib>:"Solve Linear Equations.vi"("matrix type"=Matrix_Type_of_Inverse_Matrix."General", "Known Vector"=w139, "Input Matrix"=w27) -> ("Solution Vector"=w136:dbl[])  [unwired: 1 out]
      n157 = in-place {
        w253 = 2.0 ("y")
        n158 = in-place-array #1(w136, 0, 1, 2, 3, 4, 5, 6, 7, 8, 9) -> (w252:dbl, w251:dbl, w250:dbl, w259:dbl, w257:dbl, w255:dbl, w249:dbl, w248:dbl, w247:dbl, w246:dbl)
        n159 = Divide(x=w259, y=w253) -> (x/y=w258:dbl)
        n160 = Divide(x=w257, y=w253) -> (x/y=w256:dbl)
        n161 = Divide(x=w255, y=w253) -> (x/y=w254:dbl)
        n162 = in-place-array #1(w252, w251, w250, w258, w256, w254, w249, w248, w247, w246) -> (w228:dbl[])  [unwired: 10 out]
      }
      n163 = for {
        shift-right: [w244] -> w145
        shift-left: w28 -> [w245]
        tunnel: w143 -> [w243] mode=indexing
        tunnel: w228 -> [w242] mode=indexing
        tunnel: [w242] -> w141 mode=indexing
        n164 = Insert Into Map(map in=w245, key=w243, value=w242) -> (map out=w244:map{T2, dbl})  [unwired: 2 out]
      }
    }
    frame "calc" {
      w296 = T2[][] [[enum."xx", enum."xy", enum."xw"], [enum."xy", enum."yy", enum."yw"], [enum."xw", enum."yw", enum."ww"]] items=["1", "x", "y", "xx", "xy", "yy", "xxy", "xyy", "yyy", "xxx", "xxyy", "xyyy", "xxxy", "yyyy", "xxxx", "xxz", "xyz", "yyz", "xz", "yz", "z", "wwz", "ywz", "xwz", "xxxw", "xxyw", "xyyw", "yyyw", "xxww", "xyww", "yyww", "xwww", "ywww", "wwww", "ww", "xw", "yw", "w", "wz", "xxw", "yyw", "xyw", "xww", "yww", "www"]  # aaa
      # "quadratic form"
      n165 = for {
        tunnel: w296 -> [w315] mode=indexing
        shift-right: [w313] -> w288
        shift-left: w290 -> [w314]
        tunnel: [w312] -> w297 mode=indexing
        n166 = for {
          tunnel: w315 -> [w317] mode=indexing
          shift-right: [w318] -> w313
          shift-left: w314 -> [w318]
          tunnel: [w316] -> w312 mode=indexing
          n167 = Look In Map(map=w318, key=w317) -> (value=w316:dbl)  [unwired: 1 in, 1 out]
        }
      }
      n168 = call-poly <vilib>:"Array To Matrix.vi"("Real 2D Array"=w297) -> ("Real Matrix"=w292:T5)
      n169 = for {
        tunnel: w295 -> [w310] mode=indexing
        tunnel: w294 -> [w309] mode=indexing
        tunnel: w293 -> [w308] mode=indexing
        shift-right: [w307] -> _
        shift-left: w292 -> [w307]
        tunnel: [w300] -> w291 mode=indexing
        n170 = Build Array(w310, w309, w308) -> (w306:T5)
        n171 = call-poly <vilib>:"A x B.vi"("B"=w307, "A"=w306) -> ("A x B"=w304:T5)  [unwired: 1 out]
        n172 = Transpose Matrix(1:w306) -> (0:w305:T5)
        n173 = call-poly <vilib>:"A x B.vi"("B"=w305, "A"=w304) -> ("A x B"=w311:T5)  [unwired: 1 out]
        n174 = call-poly <vilib>:"Matrix To Array.vi"("Real Matrix"=w311) -> ("Real 2D Array"=w303:dbl[][])
        n175 = Index Array(array=w303, index (row)=0, index (col)=0 ("disabled index (col)")) -> (element=w300:dbl)
      }
      n176 = call "array -- linear regression 3D -- V2.vi"("action"=array_--_fit_control_."calc", "fit map IN"=w288, "xyzw IN"=w298) -> ("fit map out"=w287:map{T2, dbl}, "xyzw OUT"=w284:T1)  [unwired: 7 in]
      n177 = Unbundle By Name(w284) -> ("z"=w286:dbl[])
      n178 = Add(x=w286, y=w291) -> (x+y=w285:dbl[])
      n179 = Bundle By Name(cluster=w284, "z"=w285) -> (w283:T1)
    }
  }
  "fit OUT" <- w22
  "fit map out" <- w12
  "xyzw OUT" <- w6
  n180 = Index Array(array=w17, index (col)=0 ("disabled index (col)")) -> ()  [unwired: 1 in, 1 out]
  n181 = Index Array(array=w21, index (col)=0 ("disabled index (col)")) -> ()  [unwired: 1 in, 1 out]
